vi "SerialMarvinSendGet.vi"(8 "error in (no error)":errorcluster, 9 "Clear Log":bool, 10 "write buffer":string="UA[3]\r\n", 11 "VISA resource name":refnum<visa-resource-name>="COM6") -> (0 "error out":errorcluster, 2 "read buffer":string)   [LabVIEW 2017]
uses:
  <vilib>/Instr/_visa.llb/VISA Configure Serial Port (Instr).vi
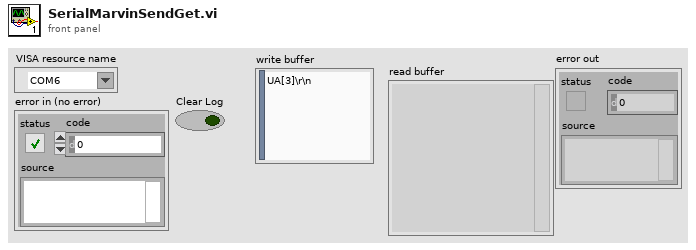
[diagram p1: front panel]
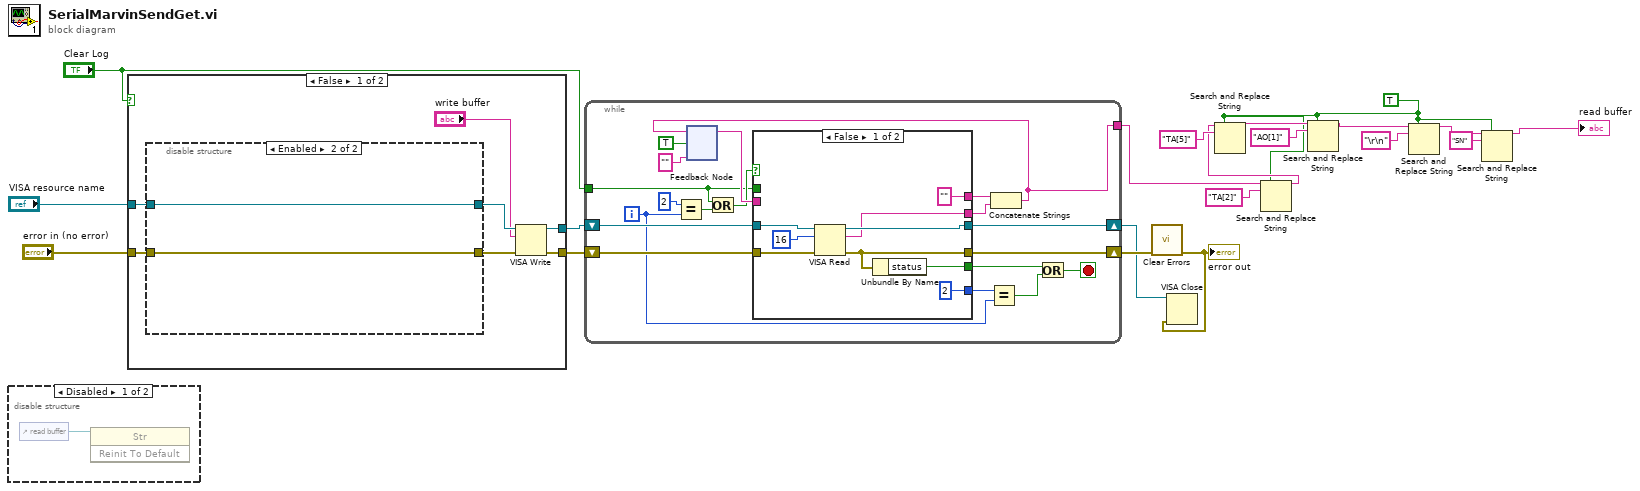
[diagram p0: block diagram]
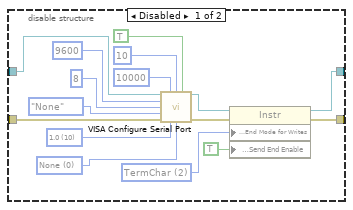
[diagram p3: hidden frame]
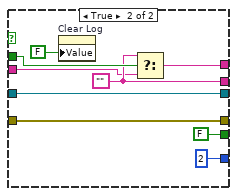
[diagram p5: hidden frame]
diagram:
  w3 = TRUE ("replace all? (F)")
  n1 = disable-structure shown="Disabled" {
    frame Disabled {
      n2 = control-ref of="read buffer"() -> (w21:refnum<vi>)
      n3 = invoke class="Str" method="Reinit To Default"(reference=w21) -> ()  [unwired: 2 in, 3 out]
    }
    frame Enabled {
    }
  }
  n4 = case shown="False" "Clear Log" {
    tunnel: "VISA resource name" -> [w28 w48]
    tunnel: "error in (no error)" -> [w27 w47]
    tunnel: [w24 w48] -> w17
    tunnel: [w23 w47] -> w16
    frame False {
      n5 = disable-structure shown="Enabled" {
        disable-tunnel: w28 -> [w44 w46]
        disable-tunnel: w27 -> [w38 w45]
        disable-tunnel: [w33 w46] -> w25
        disable-tunnel: [w32 w45] -> w26
        frame Disabled {
          w30 = u16 2 items=["None", "LastBit", "TermChar", "Break"] ("Serial Settings:Serial End Mode for Writes")
          w36 = u16 0 items=["None", "XON/XOFF", "RTS/CTS", "XON/XOFF & RTS/CTS", "DTR/DSR", "XON/XOFF & DTR/DSR"] ("flow control (0:none)")
          w37 = u16 10 items=["1.0"=10, "1.5"=15, "2.0"=20] ("stop bits (10: 1 bit)")
          n6 = call-poly "VISA Configure Serial Port"("VISA resource name"=w44, "timeout (10sec)"=u32 10000, "termination char\n(0xA = '\\n' = LF)"=u8 10 ("termination char\n(0xA = '\\n' = LF)"), "Enable Termination\nChar (T)"=TRUE ("Enable Termination\nChar (T)"), "baud rate (9600)"=u32 9600, "data bits (8)"=u16 8, "parity (0:none)"=enum16{"None", "Odd", "Even", "Mark", "Space"}."None", "error in (no error)"=w38, "stop bits (10: 1 bit)"=w37, "flow control (0:none)"=w36) -> ("VISA resource name out"=w34:refnum<visa-resource-name>, "error out"=w35:errorcluster)  [unwired: 4 in]
          n7 = property class="Instr"(reference=w34, error in=w35, "Serial Settings:End Mode for Writes"=w30, "Message Based Settings:Send End Enable"=TRUE) -> (reference out=w33:refnum<visa-resource-name>, error out=w32:errorcluster)
        }
        frame Enabled {
        }
      }
      n8 = VISA Write(VISA resource name=w25, write buffer="write buffer", error in (no error)=w26) -> (VISA resource name out=w24:refnum<visa-resource-name>, error out=w23:errorcluster)  [unwired: 1 out]
    }
    frame True {
    }
  }
  n9 = while {
    shift-right: [w67] -> w2
    shift-left: w17 -> [w63]
    shift-right: [w65] -> w20
    shift-left: w16 -> [w62]
    tunnel: [w49] -> w5
    tunnel: "Clear Log" -> [w54]
    i -> [w58]
    stop <- w50 stop-if-true
    n10 = Equal?(x=2, y=w58) -> (x = y?=w56:bool)
    n11 = feedback #1("") -> (w61:string)
    n12 = Or(x=w54, y=w56) -> (x .or. y?=w55:bool)
    n13 = case shown="False" w55 {
      tunnel: [w76 w85] -> w67
      tunnel: [w75 w79] -> w66
      tunnel: [w73 w84] -> w65
      tunnel: [w72 FALSE ("status")] -> w64
      tunnel: w63 -> [w71 w85]
      tunnel: w62 -> [w70 w84]
      tunnel: w61 -> [_ w78]
      tunnel: ["" w77] -> w60
      tunnel: [2 ("x") 2 ("x")] -> w59
      tunnel: w54 -> [_ w80]
      frame False {
        n14 = VISA Read(VISA resource name=w71, byte count=u32 16, error in (no error)=w70) -> (VISA resource name out=w76:refnum<visa-resource-name>, read buffer=w75:string, error out=w73:errorcluster)  [unwired: 1 out]
        n15 = Unbundle By Name(w73) -> ("status"=w72:bool)
      }
      frame True {
        w79 = ""
        n16 = property on="Clear Log" class="Bool (strict)"("Value"=FALSE ("Clear Log")) -> ()  [unwired: 2 in, 2 out]
        n17 = Select(t=w79, s=w80, f=w78) -> (s? t:f=w77:string)
      }
    }
    n18 = Equal?(x=w59, y=w58) -> (x = y?=w51:bool)
    n19 = Concatenate Strings(w60, w66) -> (w49:string)
    n20 = feedback-in #1(w49, TRUE) -> ()
    n21 = Or(x=w64, y=w51) -> (x .or. y?=w50:bool)
  }
  n22 = call <vilib>:"Clear Errors.vi"("error in (no error)"=w20) -> ("error out"=w1:errorcluster)  [unwired: 5 in, 1 out]
  "error out" <- w1
  n23 = VISA Close(VISA resource name=w2, error in (no error)=w1) -> ()  [unwired: 1 out]
  n24 = Search and Replace String(replace all?=w3, input string=w5, search string="TA[2]" ("substring (\"\")")) -> (result string=w4:string)  [unwired: 5 in, 3 out]
  n25 = Search and Replace String(replace all?=w3, input string=w4, search string="TA[5]" ("substring (\"\")")) -> (result string=w12:string)  [unwired: 5 in, 3 out]
  n26 = Search and Replace String(replace all?=w3, input string=w12, search string="AO[1]" ("substring (\"\")")) -> (result string=w10:string)  [unwired: 5 in, 3 out]
  n27 = Search and Replace String(replace all?=w3, input string=w10, search string="\r\n" ("substring (\"\")")) -> (result string=w9:string)  [unwired: 5 in, 3 out]
  n28 = Search and Replace String(replace all?=w3, input string=w9, search string="SN") -> (result string=→"read buffer":string)  [unwired: 5 in, 3 out]
